vi "AnimateFocusSIR.vi"() -> ()   [LabVIEW 2022 SP3]
uses:
  <vilib>/Math Plots/3D Math Plots/3D Surface/3D Surface XCtrl/3D Surface.xctl
  -AnnularRoutines/AnnularArray.ctl
  -AnnularRoutines/TransGeometry.ctl
  -AnnularRoutines/ArrayGeometry.ctl
  <vilib>/Analysis/2dsp.llb/Decimate (single shot, DBL).vi
  <vilib>/Math Plots/3D Math Plots/3D Surface/3D Surface Datatype/Public/Plot Helper (Vector).vi
  <vilib>/Utility/file.llb/Write Delimited Spreadsheet (DBL).vi
  <vilib>/Analysis/NI_AALPro.lvlib
  <vilib>/Math Plots/3D Math Plots/3D Surface/3D Surface Datatype/3D Surface Datatype.lvclass
panel:
  out "3D Surface":refnum<class "3D Plot Datatype.lvclass">[](xcontrol)
  in  "Xmt/Rcv":cluster{"XMIT":bool[], "RCV":bool[]}={"XMIT"=[TRUE, TRUE, TRUE, TRUE, TRUE], "RCV"=[TRUE, TRUE, TRUE, TRUE, TRUE]}
  out "Image Focal Depth  (cm)":dbl
  in  "start cm":dbl
  out "effective TR":i16
  out "Recip Processing":u16[][](array[ring])=[[1, 1, 1, 1, 1], [1, 1, 1, 1, 1], [1, 1, 1, 1, 1], [1, 1, 1, 1, 1], [1, 1, 1, 1, 1]] items=["0", "1", "2"]
  in  "Wave Source":T1={"Load Wave File"=FALSE, "file path"=path "E:/PVDFXducer/FiveRing/5Ring5/83micH/R1quartz.txt", "Up sample fac"=1}
  in  "kerf space (cm)":dbl=0.01 format="%.5f"
  in  "Save Path":path
  in  "Saveformat":u16(ring) items=["no save", "2D full plane", "t trace at focal plane", "6dB BWs at focus", "2D focal zones only"]
  out "file name":string
  in  "Active Annuli":bool[](array[boolean])=[TRUE, TRUE, TRUE, TRUE, TRUE, FALSE]
  in  "DR Inputs":T2 {"Tansducer" items=["F2 40 MHz", "F3 20 MHz"]}
  in  "Zones or full":u16(ring)=1 items=["full axial plots", "focal zones only"]
  in  "Calc":u16(ring)=2 items=["One way", "RT Single Rings", "R/T Full Aperture", "Time Domain PSF"]
  out "pressures":dbl[][][](array[numeric])
  in  "Center Hole":dbl format="%.2f"
  in  "Save Options":T3={"Save h Files?"=FALSE, "Save image data?"=FALSE, "Path"=path "F:/Test"}
  in  "Trans Geometry":T4={"ROC (cm)"=3.1, "a (cm)"=0.5, "focus location"=3.1} {"focus location" format="%.2f"; "a (cm)" format="%.2f"; "ROC (cm)" format="%.2f"}
  in  "Variables":T5={"#  rings"=5, "c (cm/s)"=150000, "z span (cm)"=3.0, "z steps"=10, "y span (cm)"=0.05, "y steps"=30, "time step (s)"=1e-09, "z"=0.0, "y"=0.0, "ref delay"=0.0, "freq (MHz)"=4.5, "cycles"=3.0} {"freq (MHz)" format="%.2f"; "z span (cm)" format="%.2f"; "y" format="%.2f"; "ref delay" format="%.2f"; "y span (cm)" format="%.2f"; "z" format="%.2f"; "time step (s)" format="%.2e"}
  in  "Pressure Calc":u16(ring)=1 items=["Pos Peak", "Neg peak", "Pk-Pk", "Steady State", "CW Drive", "Pii"]
  in  "# foc zones":i32=20
  # "Quantel Probe\n0 1.895 1.995 2.75 2.85 3.42  3.52  3.99 4.09  4.5 \ngeometricFocusMm=23.2\nB10 9 MHz, 7 mm OD and 27 mm focus\nB15 13 MHz, 7 mm and 23 +-2 focus"
  # "Make sure you activate elements if you increase array size."
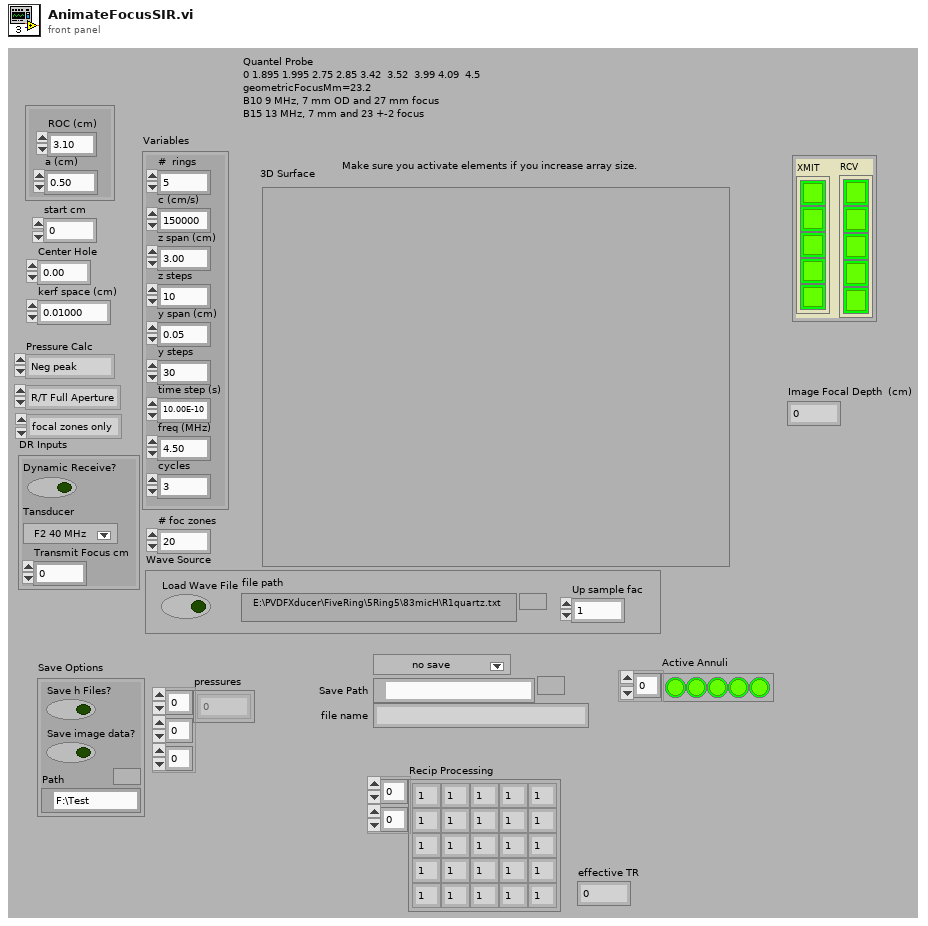
[diagram p1: front panel]
types:
  T1 = cluster{"Load Wave File":bool, "file path":path, "Up sample fac":i32}
  T2 = cluster{"Dynamic Receive?":bool, "Tansducer":u16, "Transmit Focus cm":dbl}
  T3 = cluster{"Save h Files?":bool, "Save image data?":bool, "Path":path}
  T4 = cluster{"ROC (cm)":dbl, "a (cm)":dbl, "focus location":dbl}
  T5 = cluster{"#  rings":i32, "c (cm/s)":i32, "z span (cm)":dbl, "z steps":i32, "y span (cm)":dbl, "y steps":i32, "time step (s)":sgl, "z":dbl, "y":dbl, "ref delay":dbl, "freq (MHz)":dbl, "cycles":sgl}
  T6 = typedef "AnnularArray.ctl" = cluster{"Synth Foc?":bool, "Focal Zones":i16, "Switch T/R":i16, "Trans Geometry (mm)":T7, "Sub Ap Excite?":bool, "Full Array Scan?":bool, "Xmt/Rcv":cluster{"XMIT":bool[], "RCV":bool[]}, "PulseSpacing (us)":sgl, "Xmit Ring":i32, "XMIT CHS":u8, "RCV CHS":u8, "GPU?":bool, "Save TIFF?":bool, "downfactor":i32, "RCV 1CH":u16}
  T7 = typedef "TransGeometry.ctl" = cluster{"Transducer":T8, "Geo Focus":dbl, "a (radius)":dbl, "# of rings":i32, "kerf space ":dbl, "Center Freq":dbl}
  T8 = typedef "ArrayGeometry.ctl" = u16
  T9 = cluster{"z-axis":dbl[], "y-axis":dbl[], "pressures":dbl[][]}
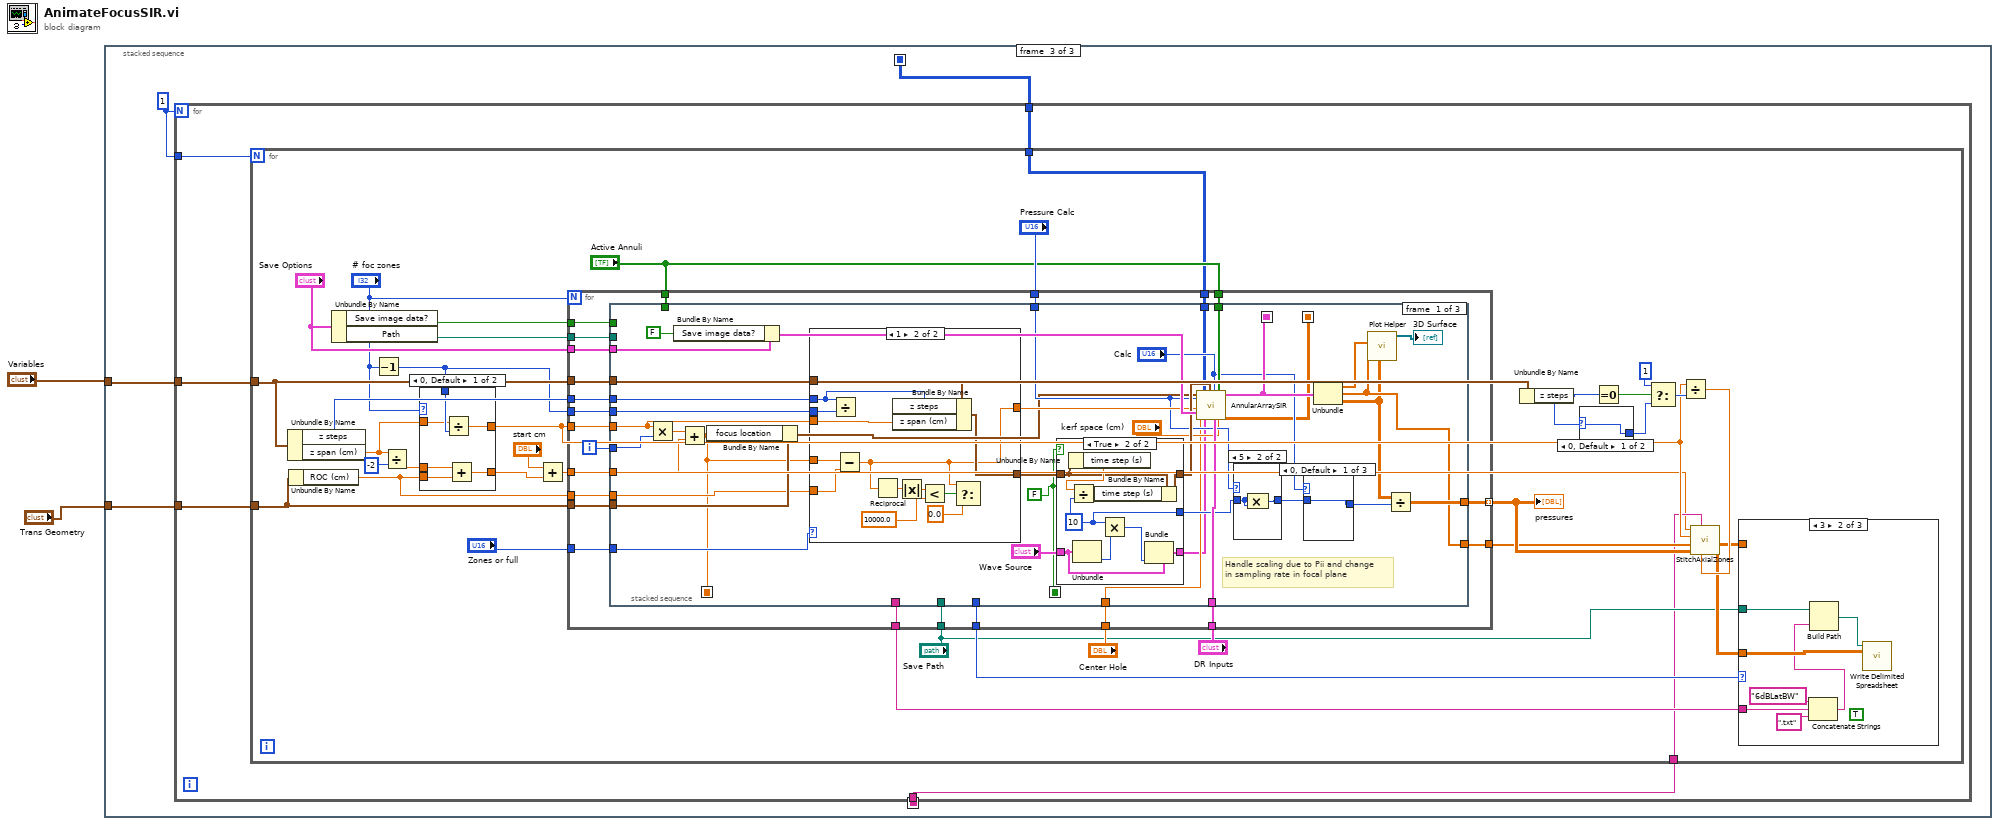
[diagram p0: block diagram]
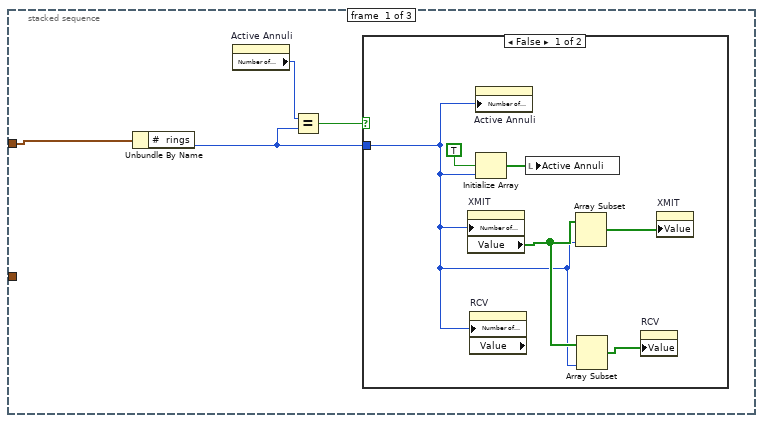
[diagram p2: hidden frame]
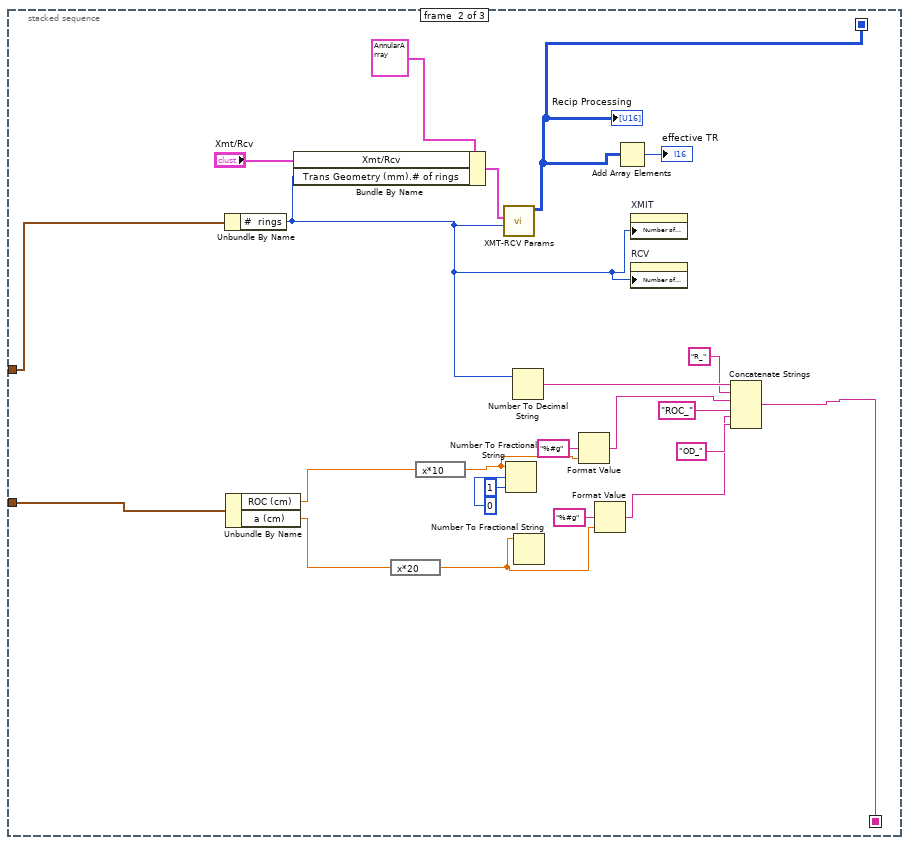
[diagram p4: hidden frame]
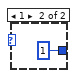
[diagram p5: hidden frame]
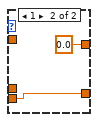
[diagram p6: hidden frame]
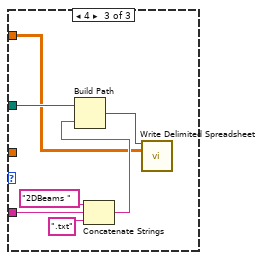
[diagram p8: hidden frame]
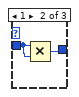
[diagram p10: hidden frame]
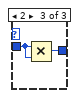
[diagram p11: hidden frame]
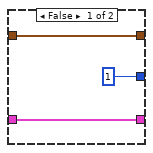
[diagram p12: hidden frame]
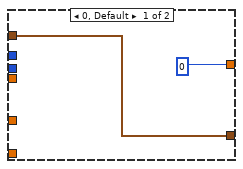
[diagram p13: hidden frame]
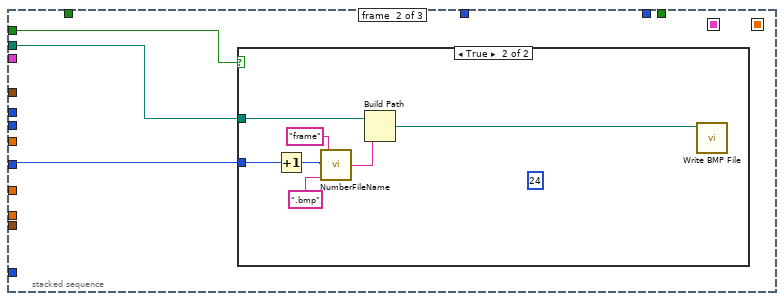
[diagram p14: hidden frame]
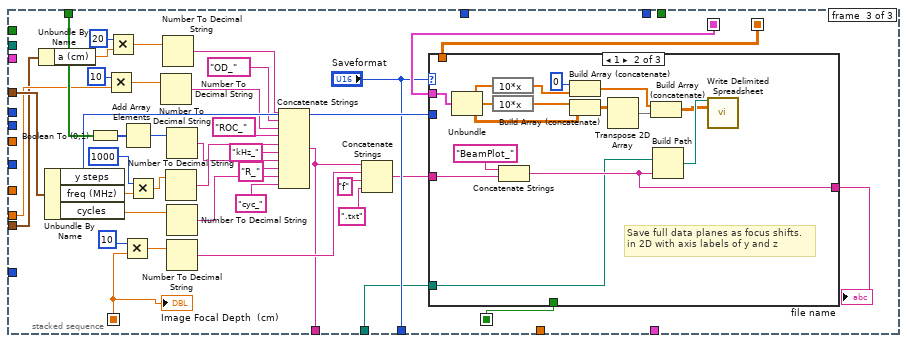
[diagram p16: hidden frame]
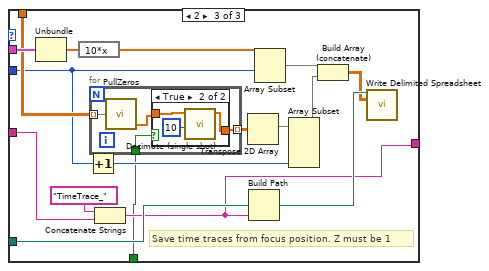
[diagram p18: hidden frame]
diagram:
  n1 = stacked-sequence {
    seq-local: [_ w34 _] -> [_ _ w38]
    seq-local: [_ w18 _] -> [_ _ w36]
    tunnel: "Variables" -> [w6 w13 w40]
    tunnel: "Trans Geometry" -> [_ w33 w37]
    frame #0 {
      n2 = Unbundle By Name(w6) -> ("#  rings"=w5:i32)
      n3 = property on="Active Annuli" class="Arr (strict)"() -> ("Number of Columns"=w4:u32)  [unwired: 2 in, 2 out]
      n4 = Equal?(x=w4, y=w5) -> (x = y?=w3:bool)
      n5 = case shown="False" w3 {
        tunnel: w5 -> [w9 _]
        frame False {
          n6 = property on="XMIT" class="Arr (strict)"("Number of Columns"=w9) -> ("Value"=w10:bool[])  [unwired: 2 in, 2 out]
          n7 = property on="RCV" class="Arr (strict)" props=["Number of Columns", "Value"]("Number of Columns"=w9) -> ()  [unwired: 2 in, 3 out]
          n8 = property on="Active Annuli" class="Arr (strict)"("Number of Columns"=w9) -> ()  [unwired: 2 in, 2 out]
          n9 = Initialize Array(TRUE, w9) -> (w11:bool[])
          n10 = local write "Active Annuli"(w11) -> ()
          n11 = Array Subset(array=w10, length=w9) -> (w8:bool[])  [unwired: 1 in]
          n12 = Array Subset(array=w10, length=w9) -> (w7:bool[])  [unwired: 1 in]
          n13 = property on="RCV" class="Arr (strict)"("Value"=w7) -> ()  [unwired: 2 in, 2 out]
          n14 = property on="XMIT" class="Arr (strict)"("Value"=w8) -> ()  [unwired: 2 in, 2 out]
        }
        frame True {
        }
      }
    }
    frame #1 {
      n15 = Unbundle By Name(w13) -> ("#  rings"=w14:i32)
      n16 = Unbundle By Name(w33) -> ("ROC (cm)"=w32:dbl, "a (cm)"=w29:dbl)
      n17 = Bundle By Name(cluster=T6 {"Synth Foc?"=FALSE, "Focal Zones"=41, "Switch T/R"=0, "Trans Geometry (mm)"={"Transducer"=0, "Geo Focus"=12.0, "a (radius)"=3.0, "# of rings"=5, "kerf space "=0.1, "Center Freq"=12.0}, "Sub Ap Excite?"=FALSE, "Full Array Scan?"=FALSE, "Xmt/Rcv"={"XMIT"=[TRUE, TRUE, TRUE, TRUE, TRUE], "RCV"=[TRUE, TRUE, TRUE, TRUE, TRUE]}, "PulseSpacing (us)"=0.0, "Xmit Ring"=0, "XMIT CHS"=0, "RCV CHS"=0, "GPU?"=FALSE, "Save TIFF?"=FALSE, "downfactor"=1, "RCV 1CH"=0} ("Ann Array Params"), "Xmt/Rcv"="Xmt/Rcv", "Trans Geometry (mm).# of rings"=w14) -> (w15:T6)
      n18 = expression code="x*20"(w29) -> (w19:dbl)
      n19 = expression code="x*10"(w32) -> (w24:dbl)
      n20 = call "XMT-RCV Params.vi"("Dig Channels"=w14, "Ann Array Params"=w15) -> ("Recip Table"=w34:i16[][])  [unwired: 4 in, 5 out]
      "Recip Processing" <- w34
      n21 = Number To Fractional String(number=w24, width (-)=i16 0, precision (6)=i16 1) -> ()  [unwired: 1 in, 1 out]
      n22 = Number To Decimal String(number=w14) -> (decimal integer string=w31:string)  [unwired: 1 in]
      n23 = Number To Fractional String(number=w19) -> ()  [unwired: 3 in, 1 out]
      n24 = Format Value(format string="%#g", value (0)=w24) -> (output string=w22:string)  [unwired: 1 in]
      n25 = Format Value(format string="%#g", value (0)=w19) -> (output string=w20:string)  [unwired: 1 in]
      n26 = Add Array Elements(numeric array=w34) -> (sum=→"effective TR":i16)
      n27 = property on="XMIT" class="Arr (strict)"("Number of Columns"=w14) -> ()  [unwired: 2 in, 2 out]
      n28 = property on="RCV" class="Arr (strict)"("Number of Columns"=w14) -> ()  [unwired: 2 in, 2 out]
      n29 = Concatenate Strings(w31, "R_" ("string"), w22, "ROC_" ("string"), w20, "OD_" ("string")) -> (w18:string)
    }
    frame #2 {
      w39 = 1
      n30 = for {
        N: w39 -> [_]
        tunnel: w40 -> [w45]
        tunnel: w38 -> [w44]
        tunnel: w39 -> [w43]
        tunnel: w37 -> [w42]
        tunnel: w36 -> [w41]
        n31 = for {
          N: w43 -> [_]
          tunnel: w45 -> [w57]
          tunnel: w44 -> [w55]
          tunnel: w42 -> [w54]
          tunnel: w41 -> [w53]
          n32 = Unbundle By Name(w57) -> ("z steps"=w72:i32, "z span (cm)"=w58:dbl)
          n33 = Unbundle By Name(w54) -> ("ROC (cm)"=w71:dbl)
          n34 = Unbundle By Name("Save Options") -> ("Save image data?"=w76:bool, "Path"=w75:path)
          n35 = Decrement(x="# foc zones") -> (x-1=w48:i32)
          n36 = Divide(x=w58, y=-2) -> (x/y=w79:dbl)
          n37 = case shown="0, Default" "# foc zones" {
            tunnel: w79 -> [w89 _]
            tunnel: w71 -> [w88 w90]
            tunnel: [w87 0.0] -> w59
            tunnel: w48 -> [w86 _]
            tunnel: w58 -> [w85 _]
            tunnel: [w84 w90] -> w52
            frame 0, Default {
              n38 = Divide(x=w85, y=w86) -> (x/y=w87:dbl)
              n39 = Add(x=w89, y=w88) -> (x+y=w84:dbl)
            }
            frame 1 {
            }
          }
          n40 = Add(x="start cm", y=w52) -> (x+y=w51:dbl)
          n41 = for {
            N: "# foc zones" -> [_]
            tunnel: w59 -> [w119]
            tunnel: w76 -> [w125]
            tunnel: "Pressure Calc" -> [w128]
            tunnel: w57 -> [w118]
            tunnel: w54 -> [w121]
            tunnel: w75 -> [w126]
            tunnel: w51 -> [w120]
            tunnel: "Center Hole" -> [w124]
            tunnel: [w123] -> w77 mode=indexing
            tunnel: "Save Options" -> [w122]
            tunnel: "Zones or full" -> [w115]
            tunnel: w72 -> [w117]
            tunnel: w48 -> [w116]
            tunnel: w71 -> [w114]
            tunnel: [w113] -> w70
            tunnel: "DR Inputs" -> [w112]
            tunnel: "Active Annuli" -> [w111]
            tunnel: "Active Annuli" -> [w110]
            tunnel: [w107] -> w60
            tunnel: [w109] -> w64
            tunnel: "Save Path" -> [w108]
            tunnel: w55 -> [w106]
            i -> [w127]
            n42 = stacked-sequence {
              seq-local: [w150 _ _] -> [_ _ w238]
              seq-local: [w134 _ _] -> [_ _ w212]
              seq-local: [w141 _ _] -> [_ _ w236]
              seq-local: [w136 _ _] -> [_ _ w235]
              tunnel: w119 -> [w157 _ _]
              tunnel: w121 -> [w166 _ w216]
              tunnel: w122 -> [w165 _ _]
              tunnel: w118 -> [w160 _ w251]
              tunnel: w128 -> [w146 _ _]
              tunnel: w127 -> [w162 w202 _]
              tunnel: w126 -> [_ w203 _]
              tunnel: w125 -> [_ w204 _]
              tunnel: w120 -> [w161 _ _]
              tunnel: w124 -> [w140 _ _]
              tunnel: [w152 _ _] -> w123
              tunnel: w117 -> [w159 _ _]
              tunnel: w116 -> [w158 _ _]
              tunnel: w115 -> [w156 _ _]
              tunnel: w114 -> [w155 _ w225]
              tunnel: [w130 _ _] -> w113
              tunnel: w112 -> [w151 _ _]
              tunnel: w111 -> [w148 _ _]
              tunnel: w110 -> [_ _ w250]
              tunnel: [_ _ "Saveformat"] -> w109
              tunnel: w108 -> [_ _ w233]
              tunnel: [_ _ w228] -> w107
              tunnel: w106 -> [w135 _ _]
              frame #0 {
                w136 = FALSE
                # "Handle scaling due to Pii and change in sampling rate in focal plane"
                n43 = Multiply(x=w157, y=w162) -> (x*y=w139:dbl)
                n44 = Bundle By Name(cluster=w165, "Save image data?"=FALSE) -> (w163:T3)
                n45 = Add(x=w139, y=w161) -> (x+y=w134:dbl)
                n46 = Bundle By Name(cluster=w166, "focus location"=w134) -> (w133:T4)
                n47 = case shown="1" w156 {
                  tunnel: [w188 w195] -> w154
                  tunnel: w160 -> [w188 w201]
                  tunnel: w159 -> [_ w196]
                  tunnel: w158 -> [_ w200]
                  tunnel: w157 -> [_ w199]
                  tunnel: [0 w189] -> w149
                  tunnel: w134 -> [_ w198]
                  tunnel: w155 -> [_ w197]
                  frame 0, Default {
                  }
                  frame 1 {
                    n48 = Divide(x=w196, y=w200) -> ()  [unwired: 1 out]
                    n49 = Subtract(x=w198, y=w197) -> (x-y=w189:dbl)
                    n50 = Reciprocal(x=w189) -> (1/x=w194:dbl)
                    n51 = Bundle By Name(cluster=w201, "z steps"=w196, "z span (cm)"=w199) -> (w195:T5)
                    n52 = Absolute Value(x=w194) -> (abs(x)=w193:dbl)
                    n53 = Less?(x=w193, y=10000.0) -> (x < y?=w191:bool)
                    n54 = Select(t=w189, s=w191, f=0.0) -> ()  [unwired: 1 out]
                  }
                }
                n55 = case shown="True" w136 {
                  tunnel: [w177 w185] -> w153
                  tunnel: w154 -> [w177 w183]
                  tunnel: [1 w182] -> w143
                  tunnel: "Wave Source" -> [w175 w179]
                  tunnel: [w175 w180] -> w137
                  frame False {
                  }
                  frame True {
                    w182 = 10
                    n56 = Unbundle By Name(w183) -> ("time step (s)"=w186:sgl)
                    n57 = Divide(x=w186, y=w182) -> (x/y=w184:sgl)
                    n58 = Unbundle(w179) -> ("Up sample fac"=w178:i32)  [unwired: 2 out]
                    n59 = Bundle By Name(cluster=w183, "time step (s)"=w184) -> (w185:T5)
                    n60 = Multiply(x=w182, y=w178) -> (x*y=w181:i32)
                    n61 = Bundle(cluster=w179, "Up sample fac"=w181) -> (w180:T1)  [unwired: 2 out]
                  }
                }
                n62 = call "AnnularArraySIR.vi"("Trans Geometry"=w133, "Pressure Calc"=w146, "center of calc"=w149, "Save Options"=w163, "Center Hole"=w140, "Recip Processing"=w135, "Wave Source"=w137, "Variables"=w153, "Calc"="Calc", "DR Inputs"=w151, "Active Annuli"=w148, "kerf space (cm)"="kerf space (cm)") -> ("Output Data"=w150:T9, "time data out"=w141:dbl[][])  [unwired: 6 in]
                n63 = case shown="5" w146 {
                  tunnel: [w167 w169] -> w145
                  tunnel: w143 -> [w167 w168]
                  frame 0, Default {
                  }
                  frame 5 {
                    n64 = Compound Arithmetic op=MULTIPLY(w168, w168) -> (w169:i32)
                  }
                }
                n65 = case shown="0, Default" "Calc" {
                  tunnel: [w170 w172 w174] -> w144
                  tunnel: w145 -> [w170 w171 w173]
                  frame 0, Default {
                  }
                  frame 1 {
                    n66 = Multiply(x=w171, y=w171) -> (x*y=w172:i32)
                  }
                  frame 2 {
                    n67 = Multiply(x=w173, y=w173) -> (x*y=w174:i32)
                  }
                }
                n68 = Unbundle(w150) -> ("z-axis"=w131:dbl[], "y-axis"=w130:dbl[], "pressures"=w129:dbl[][])
                n69 = call-poly <vilib>:"Plot Helper.vi"("z matrix"=w129, "y vector"=w130, "x vector"=w131) -> ("3D Plot lvclass Array out"=→"3D Surface":refnum<class "3D Plot Datatype.lvclass">[])  [unwired: 3 in, 5 out]
                n70 = Divide(x=w129, y=w144) -> (x/y=w152:dbl[][])
              }
              frame #1 {
                n71 = case shown="True" w204 {
                  tunnel: w203 -> [_ w206]
                  tunnel: w202 -> [_ w205]
                  frame False {
                  }
                  frame True {
                    (unwired) 24
                    n72 = Increment(x=w205) -> (x+1=w208:i32)
                    n73 = call "NumberFileName.vi"("String"=".bmp", "File number"=w208, "file name"="frame") -> ("Numbered File"=w210:string)  [unwired: 1 in]
                    n74 = Build Path(base path=w206, name or relative path=w210) -> (appended path=w207:path)
                    n75 = call <vilib>:"Write BMP File.vi"("path to BMP file"=w207) -> ()  [unwired: 5 in, 6 out]
                  }
                }
              }
              frame #2 {
                n76 = Unbundle By Name(w216) -> ("a (cm)"=w215:dbl)
                n77 = Unbundle By Name(w251) -> ("y steps"=w237:i32, "freq (MHz)"=w246:dbl, "cycles"=w249:sgl)
                n78 = Boolean To (0,1)(Boolean=w250) -> (0, 1=w248:i16[])
                n79 = Multiply(x=10, y=w225) -> (x*y=w227:dbl)
                n80 = Multiply(x=20, y=w215) -> (x*y=w218:dbl)
                n81 = Multiply(x=10, y=w212) -> (x*y=w240:dbl)
                n82 = Add Array Elements(numeric array=w248) -> (sum=w247:i16)
                n83 = Multiply(x=1000, y=w246) -> (x*y=w244:dbl)
                n84 = Number To Decimal String(number=w227) -> (decimal integer string=w224:string)  [unwired: 1 out]
                n85 = Number To Decimal String(number=w218) -> (decimal integer string=w214:string)  [unwired: 1 out]
                n86 = Number To Decimal String(number=w244) -> (decimal integer string=w222:string)  [unwired: 1 out]
                n87 = Number To Decimal String(number=w247) -> (decimal integer string=w219:string)  [unwired: 1 out]
                n88 = Number To Decimal String(number=w249) -> (decimal integer string=w243:string)  [unwired: 1 out]
                n89 = Number To Decimal String(number=w240) -> (decimal integer string=w229:string)  [unwired: 1 out]
                n90 = Concatenate Strings(w214, "OD_", w224, "ROC_", w222, "kHz_", w219, "R_", w243, "cyc_") -> (w228:string)
                n91 = Concatenate Strings(w228, w229, "f", ".txt") -> (w232:string)
                n92 = case shown="1" "Saveformat" {
                  tunnel: w238 -> [_ w267 w279]
                  tunnel: w232 -> [_ w254 w281]
                  tunnel: [_ w253 w270] -> w239
                  tunnel: w233 -> [_ w252 w280]
                  tunnel: w236 -> [_ _ w278]
                  tunnel: w237 -> [_ _ w272]
                  tunnel: w235 -> [_ _ w268]
                  frame 0, Default {
                  }
                  frame 1 {
                    # "Save full data planes as focus shifts.\nin 2D with axis labels of y and z"
                    n93 = Unbundle(w267) -> ("z-axis"=w257:dbl[], "y-axis"=w259:dbl[], "pressures"=w262:dbl[][])
                    n94 = expression code="10*x"(w257) -> (w258:dbl[])
                    n95 = expression code="10*x"(w259) -> (w256:dbl[])
                    n96 = Concatenate Strings("BeamPlot_", w254) -> (w253:string)
                    n97 = Build Array (concatenate)(0, w258) -> (w264:dbl[])
                    n98 = Build Array (concatenate)(w256, w262) -> (w265:dbl[][])
                    n99 = Transpose 2D Array(2D array=w265) -> (transposed array=w263:dbl[][])
                    n100 = Build Array (concatenate)(w264, w263) -> (w260:dbl[][])
                    n101 = Build Path(base path=w252, name or relative path=w253) -> (appended path=w261:path)
                    n102 = call-poly <vilib>:"Write Delimited Spreadsheet.vi"("file path (dialog if empty)"=w261, "2D data"=w260) -> ()  [unwired: 12 in, 2 out]
                  }
                  frame 2 {
                    # "Save time traces from focus position. Z must be 1"
                    n103 = Unbundle(w279) -> ("y-axis"=w283:dbl[])  [unwired: 2 out]
                    n104 = expression code="10*x"(w283) -> (w271:dbl[])
                    n105 = Increment(x=w272) -> (x+1=w274:i32)
                    n106 = for {
                      tunnel: w278 -> [w285] mode=indexing
                      tunnel: [w286] -> w269 mode=indexing
                      tunnel: w268 -> [w288]
                      n107 = call "PullZeros.vi"("input"=w285) -> ("output"=w287:dbl[])  [unwired: 4 out]
                      n108 = case shown="True" w288 {
                        tunnel: w287 -> [w289 w292]
                        tunnel: [w289 w291] -> w286
                        frame False {
                        }
                        frame True {
                          n109 = call-poly <vilib>:"Decimate (single shot).vi"("decimating factor"=10, "X"=w292) -> ("Decimated Array"=w291:dbl[])  [unwired: 1 in, 8 out]
                        }
                      }
                    }
                    n110 = Concatenate Strings("TimeTrace_", w281) -> (w270:string)
                    n111 = Transpose 2D Array(2D array=w269) -> (transposed array=w277:dbl[][])
                    n112 = Build Path(base path=w280, name or relative path=w270) -> (appended path=w284:path)
                    n113 = Array Subset(array=w271, index=w272) -> (w273:dbl[])  [unwired: 1 in]
                    n114 = Array Subset(array=w277, length (col)=w274) -> (w276:dbl[][])  [unwired: 3 in]
                    n115 = Build Array (concatenate)(w273, w276) -> (w275:dbl[][])
                    n116 = call-poly <vilib>:"Write Delimited Spreadsheet.vi"("file path (dialog if empty)"=w284, "2D data"=w275) -> ()  [unwired: 12 in, 2 out]
                  }
                }
                "file name" <- w239
                "Image Focal Depth  (cm)" <- w212
              }
            }
          }
          "pressures" <- w77
          n117 = Unbundle By Name(w57) -> ("z steps"=w47:i32)
          n118 = case shown="0, Default" w47 {
            selector: w47 -> [w82 _]
            tunnel: [w82 1] -> w46
            frame 0, Default {
            }
            frame 1 {
            }
          }
          n119 = Equal To 0?(x=w47) -> (x = 0?=w68:bool)
          n120 = Select(t=1, s=w68, f=w46) -> (s? t:f=w66:i32)
          n121 = Divide(x=w59, y=w66) -> (x/y=w65:dbl)
          n122 = call "StitchAxialZones.vi"("z increment axial"=w65, "FileStartName"=w53, "pressures in"=w77, "Scales"=w70, "z increment"=w59, "z Start pos"=w51) -> ("6dB data"=w63:dbl[][], "Focal zones joined"=w62:dbl[][])  [unwired: 2 out]
          n123 = case shown="3" w64 {
            tunnel: w63 -> [_ w98 _]
            tunnel: w62 -> [_ _ w99]
            tunnel: "Save Path" -> [_ w96 w104]
            tunnel: w60 -> [_ w95 w102]
            frame 0, Default {
            }
            frame 3 {
              (unwired) TRUE ("transpose? (no:F)")
              n124 = Concatenate Strings("6dBLatBW", w95, ".txt") -> (w92:string)
              n125 = Build Path(base path=w96, name or relative path=w92) -> (appended path=w94:path)
              n126 = call-poly <vilib>:"Write Delimited Spreadsheet.vi"("file path (dialog if empty)"=w94, "2D data"=w98) -> ()  [unwired: 12 in, 2 out]
            }
            frame 4 {
              n127 = Concatenate Strings("2DBeams ", w102, ".txt") -> (w103:string)
              n128 = Build Path(base path=w104, name or relative path=w103) -> (appended path=w100:path)
              n129 = call-poly <vilib>:"Write Delimited Spreadsheet.vi"("file path (dialog if empty)"=w100, "2D data"=w99) -> ()  [unwired: 12 in, 2 out]
            }
          }
        }
      }
    }
  }
